vi "Facade.vi"(0 "Data In":T5 {"IIR Filter Cluster"."Forward Coefficients" format="%.4f"; "IIR Filter Cluster"."Reverse Coefficients" format="%.4f"}, 2 "Display State In":T3, 3 "Container State":T4) -> (6 "Data Out":T5 {"IIR Filter Cluster"."Forward Coefficients" format="%.4f"; "IIR Filter Cluster"."Reverse Coefficients" format="%.4f"}, 7 "Display State Out":T3, 8 "Action":T2)   [LabVIEW 2020, in "Filter XCtl.xctl"]
uses:
  Filter XCtl.xctl
  Filter Data.ctl
  <vilib>/_xctls/Container State.ctl
  State.ctl
  <vilib>/_xctls/Action.ctl
  <vilib>/_xctls/XControlSupport.lvlib
panel:
  in  "F2":dbl caption="BW (kHz)"
  in  "Type":T1(ring) caption="Filter"
  in  "F1":dbl caption="CF (kHz)"
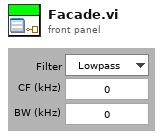
[diagram p1: front panel]
types:
  T1 = enum16{"Lowpass", "Highpass", "Bandpass", "Bandstop", "OFF"}
  T2 = typedef "XControlSupport.lvlib/Action.ctl" = cluster{"Data Changed?":bool, "State Changed?":bool, "Action Name":string}
  T3 = typedef "Filter XCtl.xctl/State.ctl" = cluster{"Show Fl/Fh?":bool}
  T4 = typedef "XControlSupport.lvlib/Container State.ctl" = cluster{"Indicator?":bool, "Run Mode?":bool, " Refnum":refnum<vi>}
  T5 = typedef "Filter XCtl.xctl/Filter Data.ctl" = cluster{"CF (kHz)":dbl, "BW (kHz)":dbl, "IIR Filter Cluster":cluster{"filter structure":enum32{"IIR 2nd Order", "IIR 4th Order"}, "Reverse Coefficients":dbl[], "Forward Coefficients":dbl[]}, "Final Filter State":dbl[], "Scale Factor":dbl, "Final Filter State 2":dbl[], "Quadrature":bool, "Type":enum16{"Lowpass", "Highpass", "Bandpass", "Bandstop", "OFF"}}
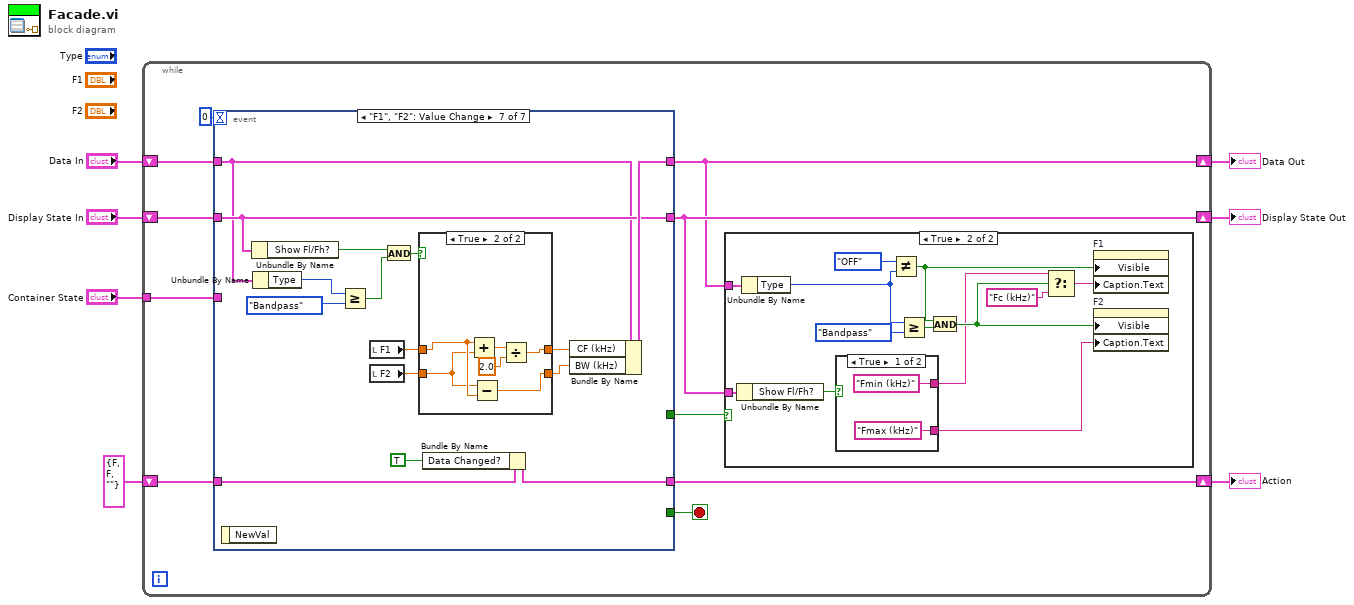
[diagram p0: block diagram]
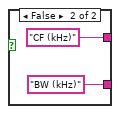
[diagram p3: hidden frame]
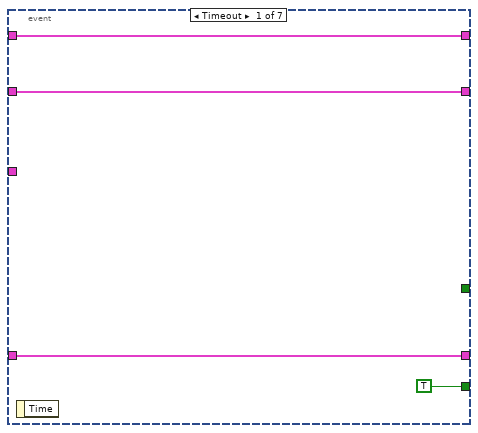
[diagram p4: hidden frame]
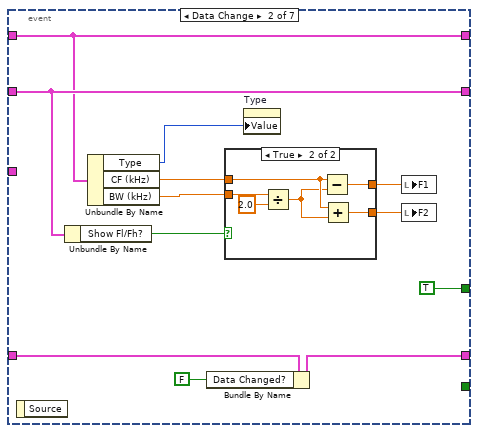
[diagram p5: hidden frame]
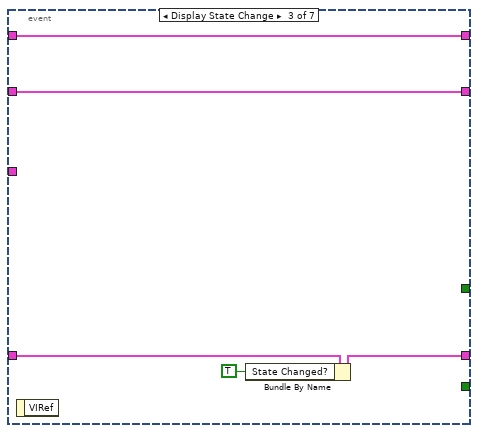
[diagram p7: hidden frame]
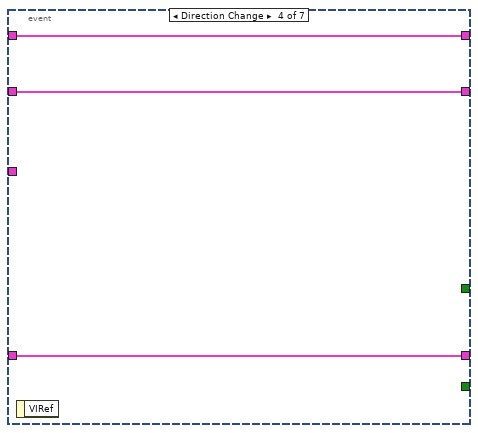
[diagram p8: hidden frame]
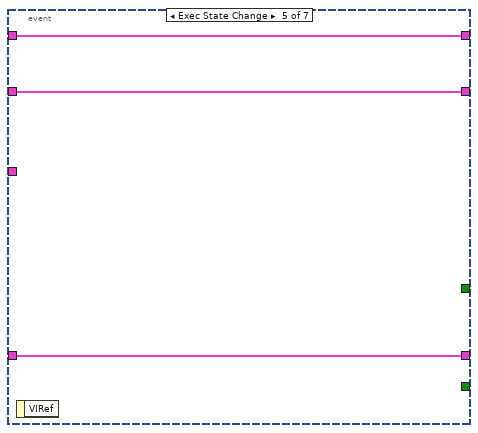
[diagram p9: hidden frame]
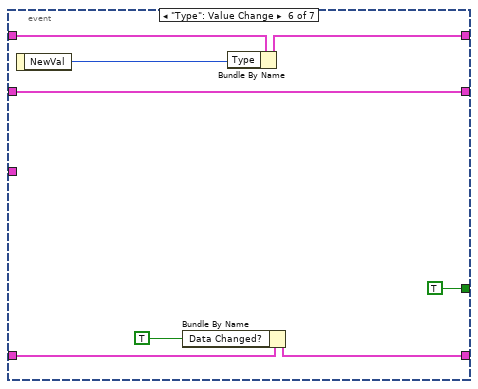
[diagram p10: hidden frame]
diagram:
  n1 = while {
    shift-right: [w10] -> w4
    shift-left: "Display State In" -> [w17]
    tunnel: "Container State" -> [w14]
    shift-right: [w9] -> w7
    shift-left: "Data In" -> [w13]
    shift-right: [w11] -> w2
    shift-left: T2 {"Data Changed?"=FALSE, "State Changed?"=FALSE, "Action Name"=""} ("Action") -> [w12]
    stop <- w16 stop-if-true
    n2 = event shown="[6] \"F1\", \"F2\": Value Change" {
      selector: _ -> [_ _ _ _ _ _ _]
      dyn-events: _ -> [_ _ _ _ _ _ _]
      timeout: 0 -> [_ _ _ _ _ _ _]
      tunnel: w17 -> [w36 w41 w61 w66 w69 w73 w88]
      tunnel: [w36 w41 w61 w66 w69 w73 w88] -> w10
      tunnel: [TRUE _ _ _ _ _ _] -> w16
      tunnel: w14 -> [_ _ _ _ _ _ _]
      tunnel: w13 -> [w35 w40 w63 w65 w68 w77 w80]
      tunnel: [w35 w40 w63 w65 w68 w76 w92] -> w9
      tunnel: [w37 w49 w60 w64 w67 w74 w89] -> w11
      tunnel: w12 -> [w37 w50 w62 w64 w67 w75 w91]
      tunnel: [_ TRUE _ _ _ TRUE _] -> w8
      event Timeout {
        n3 = event-data() -> ()  [unwired: 1 in, 1 out]
      }
      event Data Change {
        n4 = event-data() -> ()  [unwired: 1 in, 1 out]
        n5 = Unbundle By Name(w41) -> ("Show Fl/Fh?"=w47:bool)
        n6 = Unbundle By Name(w40) -> ("Type"=w42:T1, "CF (kHz)"=w46:dbl, "BW (kHz)"=w44:dbl)
        n7 = Bundle By Name(cluster=w50, "Data Changed?"=FALSE) -> (w49:T2)
        n8 = case shown="True" w47 {
          tunnel: w46 -> [w52 w55]
          tunnel: [w52 w56] -> w45
          tunnel: [w51 w53] -> w43
          tunnel: w44 -> [w51 w58]
          frame False {
          }
          frame True {
            n9 = Divide(x=w58, y=2.0) -> (x/y=w54:dbl)
            n10 = Subtract(x=w55, y=w54) -> (x-y=w56:dbl)
            n11 = Add(x=w55, y=w54) -> (x+y=w53:dbl)
          }
        }
        n12 = property on="Type" class="Enum (strict)"("Value"=w42) -> ()  [unwired: 2 in, 2 out]
        n13 = local write "F1"(w45) -> ()
        n14 = local write "F2"(w43) -> ()
      }
      event Display State Change {
        n15 = event-data() -> ()  [unwired: 1 in, 1 out]
        n16 = Bundle By Name(cluster=w62, "State Changed?"=TRUE) -> (w60:T2)
      }
      event Direction Change {
        n17 = event-data() -> ()  [unwired: 1 in, 1 out]
      }
      event Exec State Change {
        n18 = event-data() -> ()  [unwired: 1 in, 1 out]
      }
      event "Type": Value Change {
        n19 = event-data() -> ("NewVal"=w72:T1)  [unwired: 1 in]
        n20 = Bundle By Name(cluster=w75, "Data Changed?"=TRUE) -> (w74:T2)
        n21 = Bundle By Name(cluster=w77, "Type"=w72) -> (w76:T5)
      }
      event "F1", "F2": Value Change {
        n22 = event-data() -> ()  [unwired: 1 in, 1 out]
        n23 = Unbundle By Name(w88) -> ("Show Fl/Fh?"=w83:bool)
        n24 = Unbundle By Name(w80) -> ("Type"=w81:T1)
        n25 = Greater Or Equal?(x=w81, y=T1."Bandpass") -> (x >= y?=w78:bool)
        n26 = local read "F1"() -> (w87:dbl)
        n27 = local read "F2"() -> (w85:dbl)
        n28 = And(x=w83, y=w78) -> (x .and. y?=w79:bool)
        n29 = case shown="True" w79 {
          tunnel: w87 -> [w94 w97]
          tunnel: [w94 w99] -> w86
          tunnel: [w93 w95] -> w84
          tunnel: w85 -> [w93 w96]
          frame False {
          }
          frame True {
            n30 = Add(x=w97, y=w96) -> (x+y=w100:dbl)
            n31 = Subtract(x=w96, y=w97) -> (x-y=w95:dbl)
            n32 = Divide(x=w100, y=2.0) -> (x/y=w99:dbl)
          }
        }
        n33 = Bundle By Name(cluster=w91, "Data Changed?"=TRUE) -> (w89:T2)
        n34 = Bundle By Name(cluster=w80, "CF (kHz)"=w86, "BW (kHz)"=w84) -> (w92:T5)
      }
    }
    n35 = case shown="True" w8 {
      tunnel: w10 -> [_ w19]
      tunnel: w9 -> [_ w18]
      frame False {
      }
      frame True {
        n36 = Unbundle By Name(w19) -> ("Show Fl/Fh?"=w22:bool)
        n37 = Unbundle By Name(w18) -> ("Type"=w23:T1)
        n38 = case shown="True" w22 {
          tunnel: ["Fmin (kHz)" "CF (kHz)"] -> w25
          tunnel: ["Fmax (kHz)" "BW (kHz)"] -> w20
          frame True {
          }
          frame False {
          }
        }
        n39 = Not Equal?(x=T1."OFF" ("y"), y=w23) -> (x != y?=w28:bool)
        n40 = Greater Or Equal?(x=w23, y=T1."Bandpass") -> (x >= y?=w29:bool)
        n41 = And(x=w28, y=w29) -> (x .and. y?=w27:bool)
        n42 = Select(t=w25, s=w27, f="Fc (kHz)" ("t")) -> (s? t:f=w26:string)
        n43 = property on="F1" class="DigNum (strict)"("Visible"=w28, "Caption.Text"=w26) -> ()  [unwired: 2 in, 2 out]
        n44 = property on="F2" class="DigNum (strict)"("Visible"=w27, "Caption.Text"=w20) -> ()  [unwired: 2 in, 2 out]
      }
    }
  }
  "Display State Out" <- w4
  "Data Out" <- w7
  "Action" <- w2
